vi "Read Color Pair.vi"(8 "error in (no error)":errorcluster, 9 "Active Plot":i32, 11 "3D Bar in":refnum<class "3D Bar.lvclass">) -> (0 "error out":errorcluster, 2 "Color Pair Array":cluster{"Color":u32, "String":string}[](array[cluster]), 3 "3D Bar out":refnum<class "3D Bar.lvclass">)   [LabVIEW 2017, in "3D Bar.lvclass"]
uses:
  <vilib>/Math Plots/3D Math Plots/3D Bar/3D Bar/3D Bar.lvclass
  <vilib>/Math Plots/3D Math Plots/3D Bar/3D Bar/3D Bar.lvclass/3D Bar.ctl
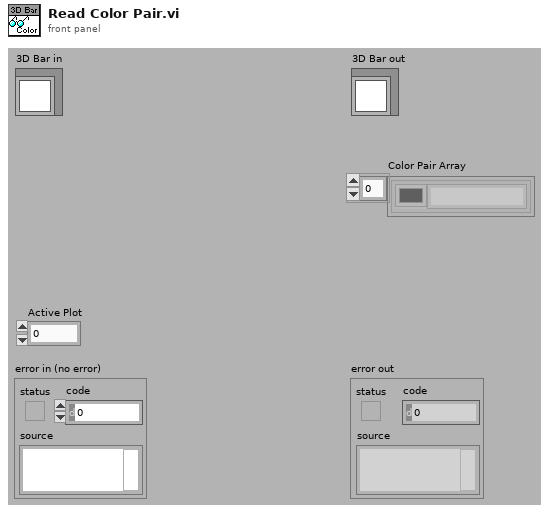
[diagram p1: front panel]
types:
  T1 = typedef "3D Bar.lvclass/3D Bar Property Array.ctl" = T2[]
  T2 = typedef "3D Bar.lvclass/3D Bar Property.ctl" = cluster{"General Property":cluster{"Plot Name":string, "Coordinate System":enum16{"Cartesian", "Cylindrical", "Spherical"}, "Opacity":sgl}, "Projection Property":cluster{"Draw XY":bool, "Draw YZ":bool, "Draw XZ":bool}, "Plot Property":cluster{"Line Style":T3, "Line Width":sgl, "Line Color":u32, "Antialiasing":bool}, "Bar Property":cluster{"Bar Mode":enum16{"Detach", "Group", "Stack"}, "Bar Width":sgl, "Color Pair Array":cluster{"Color":u32, "String":string}[]}}
  T3 = typedef "3D Plot.lvclass/Line Type.ctl" = enum16{"None", "Solid", "Dash", "Dot", "Dash Dot"}
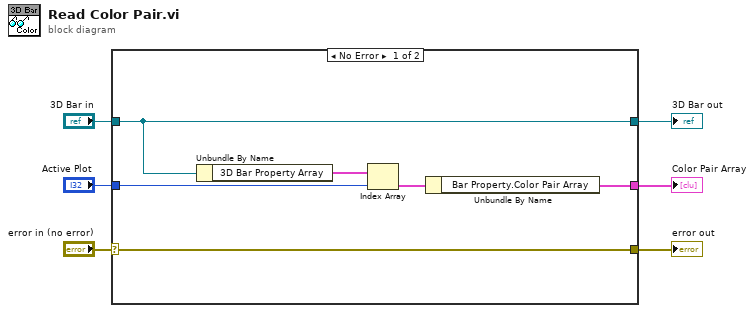
[diagram p0: block diagram]
diagram:
  n1 = case shown="No Error" "error in (no error)" {
    selector: "error in (no error)" -> [w12 w14]
    tunnel: "3D Bar in" -> [w11 w13]
    tunnel: [w11 w13] -> w1
    tunnel: [w12 w14] -> w3
    tunnel: "Active Plot" -> [w9 _]
    tunnel: [w7 _] -> w2
    frame No Error {
      n2 = Unbundle By Name(w11) -> ("3D Bar Property Array"=w10:T1)
      n3 = Index Array(array=w10, index=w9) -> (element=w8:T2)
      n4 = Unbundle By Name(w8) -> ("Bar Property.Color Pair Array"=w7:cluster{"Color":u32, "String":string}[])
    }
    frame Error {
    }
  }
  "error out" <- w3
  "3D Bar out" <- w1
  "Color Pair Array" <- w2
